vi "Destroy.vi"(0 "reference in":refnum<class "DQMHModuleNode.lvclass">, 5 "error in (no error)":errorcluster) -> (14 "reference out":refnum<class "DQMHModuleNode.lvclass">, 19 "error out":errorcluster)   [LabVIEW 2020, in "DQMHModuleNode.lvclass"]
doc: "Destroys a ClassNode object created with a ClassNode constructor VI.\n\n[GOOP 2.1]"
uses:
  <resource>/Framework/Providers/Open_GDS/UML/DQMHModuleNode_class/DQMHModuleNode.lvclass
  <resource>/Framework/Providers/Open_GDS/UML/RectangularNode_class/RectangularNode.lvclass
  <resource>/Framework/Providers/Open_GDS/UML/MultiLineString_class/MultiLineString.lvclass
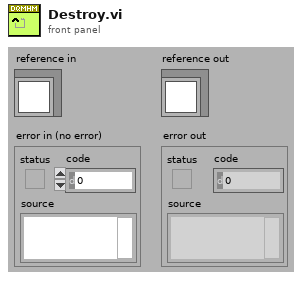
[diagram p1: front panel]
types:
  T1 = typedef "DQMHModuleNode.lvclass/ObjectAttributes.ctl" = cluster{"DescriptionHeight":dbl, "InternalDataHeight":dbl, "EventsHeight":dbl, "Name":refnum<class "MultiLineString.lvclass">, "Description":refnum<class "MultiLineString.lvclass">, "InternalData":refnum<class "MultiLineString.lvclass">, "Events":refnum<class "MultiLineString.lvclass">, "showDescription":bool, "showInternalData":bool, "showEvents":bool, "DEFAULT_ROUNDING":i32, "DEFAULT_WIDTH":i32, "DEFAULT_HEIGHT":i32, "ClassPath":path, "Template":string, "Icon":u8[][]}
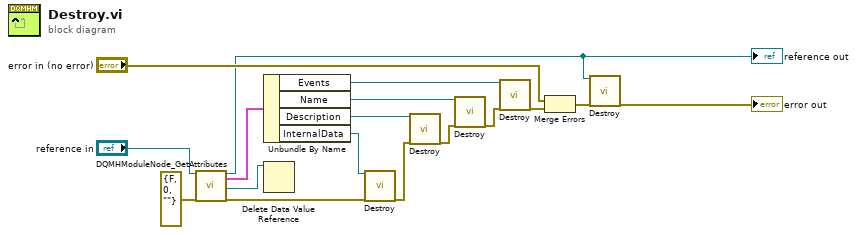
[diagram p0: block diagram]
diagram:
  n1 = call <resource>:"DQMHModuleNode_GetAttributes.vi"("reference in"="reference in", "error in (no error)"=errorcluster {"status"=FALSE, "code"=0, "source"=""}) -> ("reference out"=w7:refnum<class "DQMHModuleNode.lvclass">, "Data"=w5:T1, "DataRef"=w4:refnum<data-value>, "error out"=w10:errorcluster)  [unwired: 1 in, 13 out]
  "reference out" <- w7
  n2 = Unbundle By Name(w5) -> ("Events"=w1:refnum<class "MultiLineString.lvclass">, "Name"=w11:refnum<class "MultiLineString.lvclass">, "Description"=w12:refnum<class "MultiLineString.lvclass">, "InternalData"=w13:refnum<class "MultiLineString.lvclass">)
  n3 = Delete Data Value Reference(data value reference=w4) -> ()  [unwired: 1 in, 2 out]
  n4 = call-dynamic "Destroy.vi"("reference"=w13, "error in (no error)"=w10) -> ("error out"=w9:errorcluster)  [unwired: 16 in, 1 out]
  n5 = call-dynamic "Destroy.vi"("reference"=w12, "error in (no error)"=w9) -> ("error out"=w8:errorcluster)  [unwired: 16 in, 1 out]
  n6 = call-dynamic "Destroy.vi"("reference"=w11, "error in (no error)"=w8) -> ("error out"=w3:errorcluster)  [unwired: 16 in, 1 out]
  n7 = call-dynamic "Destroy.vi"("reference"=w1, "error in (no error)"=w3) -> ("error out"=w2:errorcluster)  [unwired: 16 in, 1 out]
  n8 = Merge Errors("error in (no error)", w2) -> (w6:errorcluster)
  n9 = call-parent "Destroy.vi"("reference"=w7, "error in (no error)"=w6) -> ("error out"=→"error out":errorcluster)  [unwired: 16 in, 1 out]
